vi "LVClass_HasoData Get Info.vi"(0 "HasoData in":refnum<class "HasoData.lvclass">, 11 "error in (no error)":errorcluster) -> (4 "HasoData out":refnum<class "HasoData.lvclass">, 8 "DataHaso acquisition information":T1 {"HASO information"."Lower calibration wavelength (nm)" min=0.0 max=1.0; "SLOPES ENGINE information"."Pupil average" min=0.0 max=1.0}, 15 "error out":errorcluster)   [LabVIEW 2020, in "HasoData.lvclass"]
doc: "Get informations from HasoData object.\n\n<B>HasoDataIn</B> : HasoData object.\n<B>HasoDataOut</B> : HasoData object.\n<B>haso_model</B> : Sensor model.\n<B>haso_serial_number</B> : Haso serial number.\n<B>camera_serial_number</B> : Camera serial number.\n<B>revisions</B> : Revision number.\n<B>lower_calibration_wl</B> : Lower calibration wavelength (nm).\n<B>upper_calibration_wl</B> : Upper calibration wavelength (nm).\n<B>exposure_time_requested</B> : Exposure duration requested, in microsecond.\n<B>exposure_time_applied</B> : Exposure duration applied, in microsecond.\n<B>nb_summed_images</B> : Number of summed images.\n<B>time_stamp</B> : Timestamp.\n<B>is_background_removed</B> : Background removed value.\n<B>is_smearing_removed</B> : Smearing removed value.\n<B>wavelength_nm</B> : Source wavelength (nm).\n<B>session_name</B> : Session name.\n<B>trigger_type</B> : Trigger mode.\n<B>comments</B> : Comments.\n<B>max_level</B> : Max level value.\n<B>start_subpupil</B> : Start subpupil position (um)\n<B>denoising_strength</B> : Sensitivity of spot detection (between 0 and 1). Modulates noise management\n when computing slopes on summed images.\n * 0 : Release constraint on noise to detect as much sub-pupils as possible.\n * 1 : Do not take into account the noise reduction caused by summing.\n<B>ErrorIn </B> : Error\n<B>ErrorOut </B> : Error"
uses:
  HasoData.lvclass
  DataHaso acquisition information.ctl
  HASO information.ctl
  Image information.ctl
  Image general information.ctl
  Image acquisition information.ctl
  Point2D.ctl
  Data alignment enum.ctl
  SlopesEngineSetup.ctl
  HasoData.lvclass/HasoData.ctl
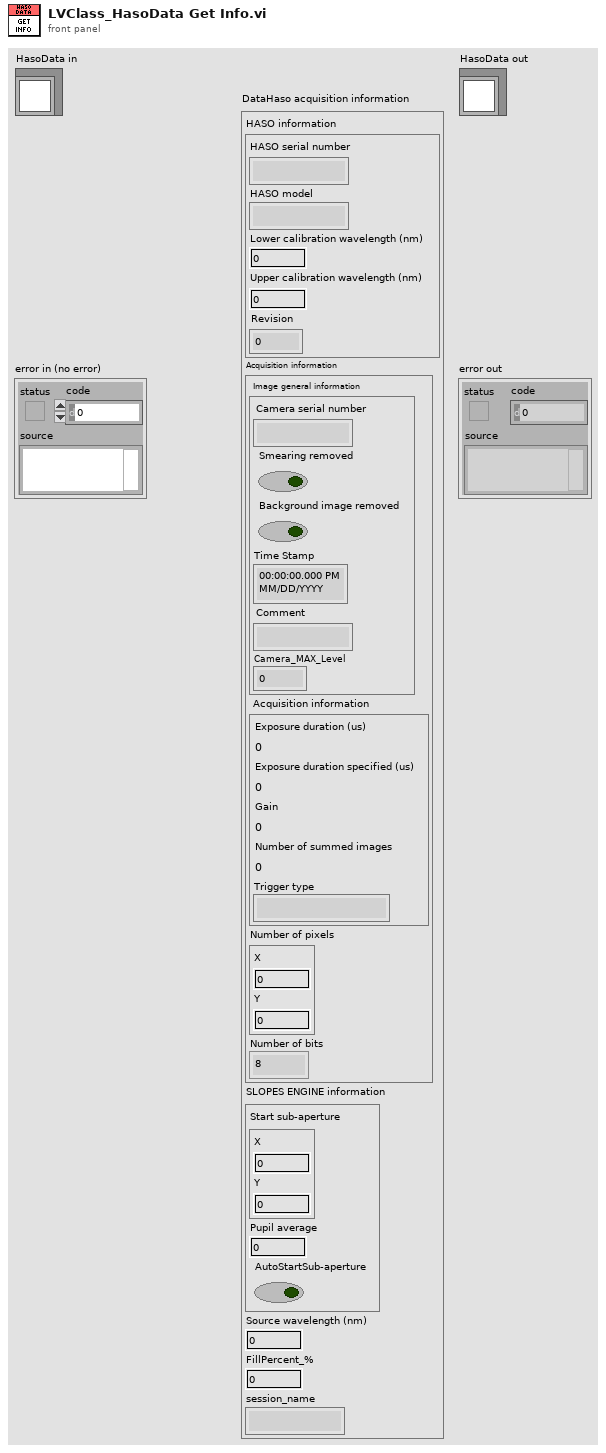
[diagram p1: front panel]
types:
  T1 = typedef "DataHaso acquisition information.ctl" = cluster{"HASO information":T2, "Acquisition information":T3, "SLOPES ENGINE information":T8, "Source wavelength (nm)":dbl, "FillPercent_%":dbl, "session_name":string}
  T2 = typedef "HASO information.ctl" = cluster{"HASO serial number":string, "HASO model":string, "Lower calibration wavelength (nm)":dbl, "Upper calibration wavelength (nm)":dbl, "Revision":i32}
  T3 = typedef "Image information.ctl" = cluster{"Image general information":T4, "Acquisition information":T5, "Number of pixels":T6, "Number of bits":T7}
  T4 = typedef "Image general information.ctl" = cluster{"Camera serial number":string, "Smearing removed":bool, "Background image removed":bool, "Time Stamp":timestamp, "Comment":string, "Camera_MAX_Level":i32}
  T5 = typedef "Image acquisition information.ctl" = cluster{"Exposure duration (us)":i32, "Exposure duration specified (us)":i32, "Gain":sgl, "Number of summed images":i32, "Trigger type":string}
  T6 = typedef "Point2D.ctl" = cluster{"X":u32, "Y":u32}
  T7 = typedef "Data alignment enum.ctl" = enum16{"8", "16", "32"}
  T8 = typedef "SlopesEngineSetup.ctl" = cluster{"Start sub-aperture":T6, "Pupil average":dbl, "AutoStartSub-aperture":bool}
  T9 = typedef "ClassID.ctl" = i64
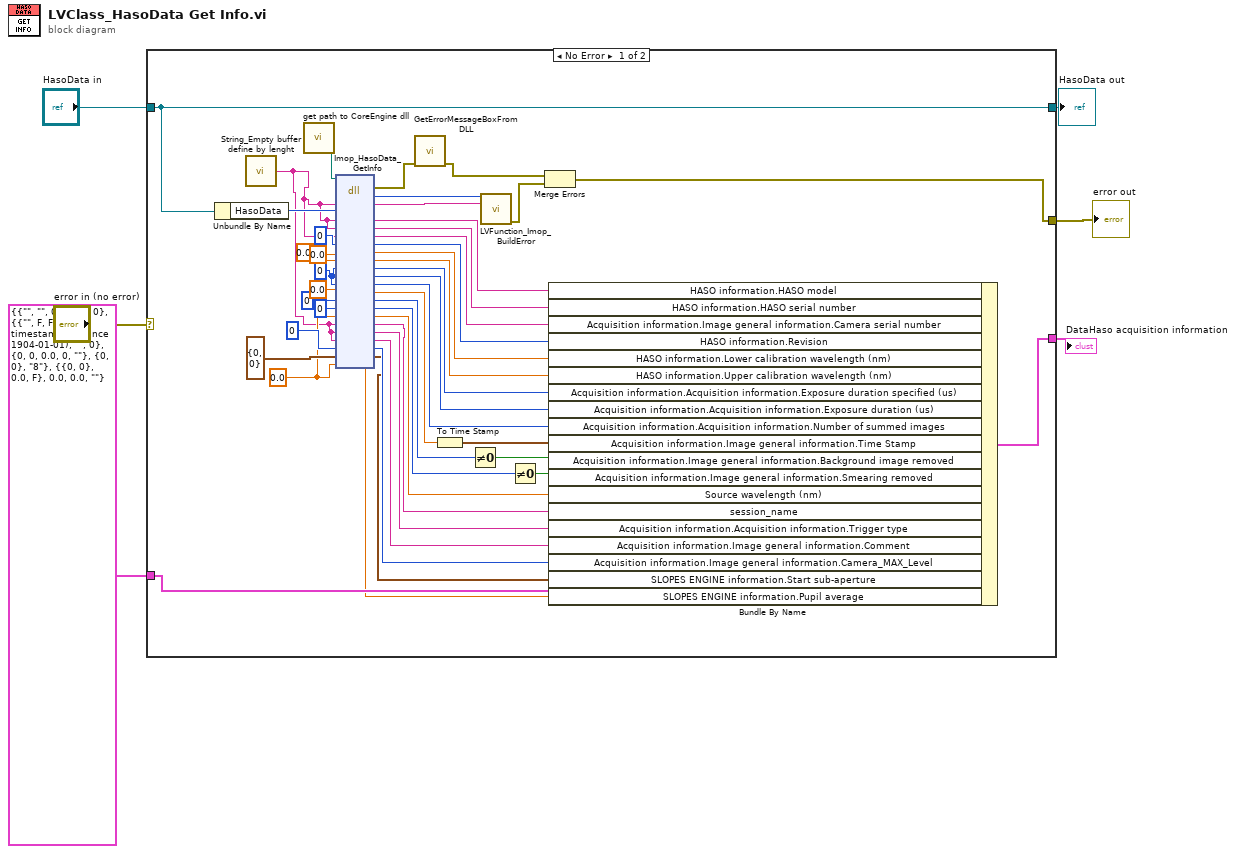
[diagram p0: block diagram]
diagram:
  n1 = case shown="No Error" "error in (no error)" {
    selector: "error in (no error)" -> [_ w52]
    tunnel: [w26 w52] -> w4
    tunnel: [w46 w51] -> w3
    tunnel: "HasoData in" -> [w46 w51]
    tunnel: [w30 _] -> w2
    tunnel: T1 {"HASO information"={"HASO serial number"="", "HASO model"="", "Lower calibration wavelength (nm)"=0.0, "Upper calibration wavelength (nm)"=0.0, "Revision"=0}, "Acquisition information"={"Image general information"={"Camera serial number"="", "Smearing removed"=FALSE, "Background image removed"=FALSE, "Time Stamp"=timestamp(0 s since 1904-01-01), "Comment"="", "Camera_MAX_Level"=0}, "Acquisition information"={"Exposure duration (us)"=0, "Exposure duration specified (us)"=0, "Gain"=0.0, "Number of summed images"=0, "Trigger type"=""}, "Number of pixels"={"X"=0, "Y"=0}, "Number of bits"=enum."8"}, "SLOPES ENGINE information"={"Start sub-aperture"={"X"=0, "Y"=0}, "Pupil average"=0.0, "AutoStartSub-aperture"=FALSE}, "Source wavelength (nm)"=0.0, "FillPercent_%"=0.0, "session_name"=""} ("DataHaso acquisition information 2") -> [w29 _]
    frame No Error {
      w11 = 0.0 ("Pupil average")
      w41 = u32 0 ("ExposureTimeOrder")
      n2 = Unbundle By Name(w46) -> ("HasoData"=w45:T9)
      n3 = call "String_Empty buffer define by lenght.vi"() -> ("Empty buffer"=w7:string)  [unwired: 1 in]
      n4 = call "get path to CoreEngine dll.vi"() -> ("path to wavekit library"=w48:path)  [unwired: 14 in, 1 out]
      n5 = dll-call lib="D:/soft/HASO_v3/SVN_trunk/ImOpCoreEngine4_LV2011/DLLs/c_interface_vc100.dll" fn="Imop_HasoData_GetInfo"(path in=w48, "message"=w7, "HasoData"=w45, "HasoModel"=w7, "HasoSerial Number"=w7, "CameraSerialNumber"=w7, "Revision"=u32 0, "LowerCalibrationWl"=0.0, "UpperCalibrationWl"=0.0, "ExposureTimeOrder"=w41, "ExposureTimeState"=w41, "NbSummedImages"=w41, "TimeStamp"=0.0, "BackgroundRemoved"=u8 0, "Smearing_Removed"=u8 0, "wavelength_nm"=w11, "session_name"=w7, "TriggerType"=w7, "comments"=w7, "MaxLevel"=u64 0, "StartSubPupil"=T6 {"X"=0, "Y"=0} ("Size"), "Pupil average"=w11) -> (error out=w47:errorcluster, "return type"=w50:i32, "message"=w49:string, "HasoModel"=w39:string, "HasoSerial Number"=w8:string, "CameraSerialNumber"=w17:string, "Revision"=w38:u32, "LowerCalibrationWl"=w37:dbl, "UpperCalibrationWl"=w36:dbl, "ExposureTimeOrder"=w35:u32, "ExposureTimeState"=w34:u32, "NbSummedImages"=w33:u32, "TimeStamp"=w32:dbl, "BackgroundRemoved"=w21:u8, "Smearing_Removed"=w19:u8, "wavelength_nm"=w10:dbl, "session_name"=w9:string, "TriggerType"=w16:string, "comments"=w15:string, "MaxLevel"=w18:u64, "StartSubPupil"=w13:T6, "Pupil average"=w12:dbl)  [unwired: 3 in, 1 out]
      n6 = call "GetErrorMessageBoxFromDLL.vi"("error IN"=w47) -> ("error OUT"=w28:errorcluster)  [unwired: 10 in]
      n7 = To Time Stamp(1:w32) -> (0:w31:timestamp)
      n8 = Not Equal To 0?(x=w21) -> (x != 0?=w22:bool)
      n9 = call "LVFunction_Imop_BuildError.vi"("code"=w50, "String to Prepend to source (\"\")"=w49) -> ("error out"=w27:errorcluster)  [unwired: 13 in]
      n10 = Not Equal To 0?(x=w19) -> (x != 0?=w20:bool)
      n11 = Merge Errors(w28, w27) -> (w26:errorcluster)
      n12 = Bundle By Name(cluster=w29, "HASO information.HASO model"=w39, "HASO information.HASO serial number"=w8, "Acquisition information.Image general information.Camera serial number"=w17, "HASO information.Revision"=w38, "HASO information.Lower calibration wavelength (nm)"=w37, "HASO information.Upper calibration wavelength (nm)"=w36, "Acquisition information.Acquisition information.Exposure duration specified (us)"=w35, "Acquisition information.Acquisition information.Exposure duration (us)"=w34, "Acquisition information.Acquisition information.Number of summed images"=w33, "Acquisition information.Image general information.Time Stamp"=w31, "Acquisition information.Image general information.Background image removed"=w22, "Acquisition information.Image general information.Smearing removed"=w20, "Source wavelength (nm)"=w10, "session_name"=w9, "Acquisition information.Acquisition information.Trigger type"=w16, "Acquisition information.Image general information.Comment"=w15, "Acquisition information.Image general information.Camera_MAX_Level"=w18, "SLOPES ENGINE information.Start sub-aperture"=w13, "SLOPES ENGINE information.Pupil average"=w12) -> (w30:T1)
    }
    frame Error {
    }
  }
  "error out" <- w4
  "HasoData out" <- w3
  "DataHaso acquisition information" <- w2
